vi "init_round_buoy.vi"(9 "Mission.lvclass":refnum<class "Mission.lvclass">, 11 "Buoy to Round":T1 {"North" format="%#_10f"; "East" format="%#_8f"}) -> (3 "Mission out":refnum<class "Mission.lvclass">)   [LabVIEW 2011, in "Mission.lvclass"]
uses:
  Mission.lvclass
  2 Typedefs/UTM Location.ctl
  Mission.lvclass/Mission.ctl
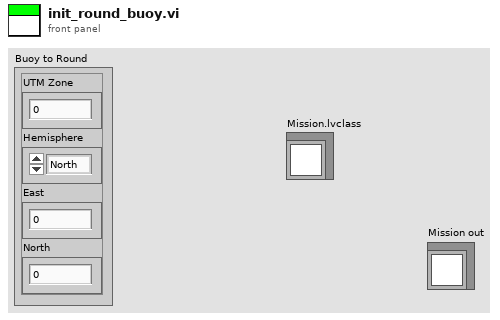
[diagram p1: front panel]
types:
  T1 = typedef "UTM Location.ctl" = cluster{"UTM Zone":dbl, "Hemisphere":enum16{"North", "South"}, "East":dbl, "North":dbl}
  T2 = enum16{"Round Buoy", "Drive", "Pass Buoys", "Station Keeping"}
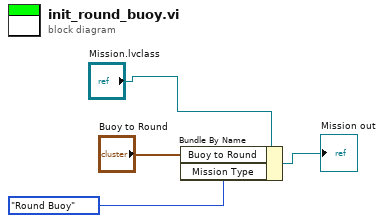
[diagram p0: block diagram]
diagram:
  n1 = Bundle By Name(cluster="Mission.lvclass", "Buoy to Round"="Buoy to Round", "Mission Type"=T2."Round Buoy") -> (→"Mission out":refnum<class "Mission.lvclass">)
